vi "Facade.vi"(0 "Data In":T6, 2 "Display State In":T2, 3 "Container State":T5) -> (6 "Data Out":T6, 7 "Display State Out":T2, 8 "Action":T1)   [LabVIEW 2012, in "Hover Button.xctl"]
doc: "This facade vi is just a boolean button. The functionality associated with it allows the color properties of the button to change depending on whether the mouse is 'hovering' on the button."
uses:
  Hover Button.xctl
  Data.ctl
  <vilib>/_xctls/Container State.ctl
  State.ctl
  Button Colors.ctl
  Font Properties.ctl
  <vilib>/_xctls/Action.ctl
  Color Select.ctl
  <vilib>/_xctls/XControlSupport.lvlib
panel:
  in  "Boolean":bool
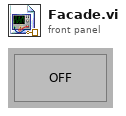
[diagram p1: front panel]
types:
  T1 = typedef "XControlSupport.lvlib/Action.ctl" = cluster{"Data Changed?":bool, "State Changed?":bool, "Action Name":string}
  T2 = typedef "Hover Button.xctl/State.ctl" = cluster{"On Text":string, "Off Text":string, "Current Color":T3, "Button Color":T3, "Hover Color":T3, "Show Boolean Text":bool, "Multiple Strings":bool, "Font":T4}
  T3 = typedef "Hover Button.xctl/Button Colors.ctl" = cluster{"On Color":u32, "Text Color":u32, "Off Color":u32}
  T4 = typedef "Hover Button.xctl/Font Properties.ctl" = cluster{"Font Name":string, "Size":u32, "Bold":bool, "Italic":bool, "Underline":bool, "Strikeout":bool, "Alignment":enum16{"Left", "Center", "Right"}}
  T5 = typedef "XControlSupport.lvlib/Container State.ctl" = cluster{"Indicator?":bool, "Run Mode?":bool, " Refnum":refnum<vi>}
  T6 = typedef "Hover Button.xctl/Data.ctl" = bool
  T7 = typedef "Hover Button.xctl/Color Select.ctl" = enum16{"Current Color", "Button Color", "Hover Color"}
  T8 = cluster{"Text Color":u32, "Background Color":u32}
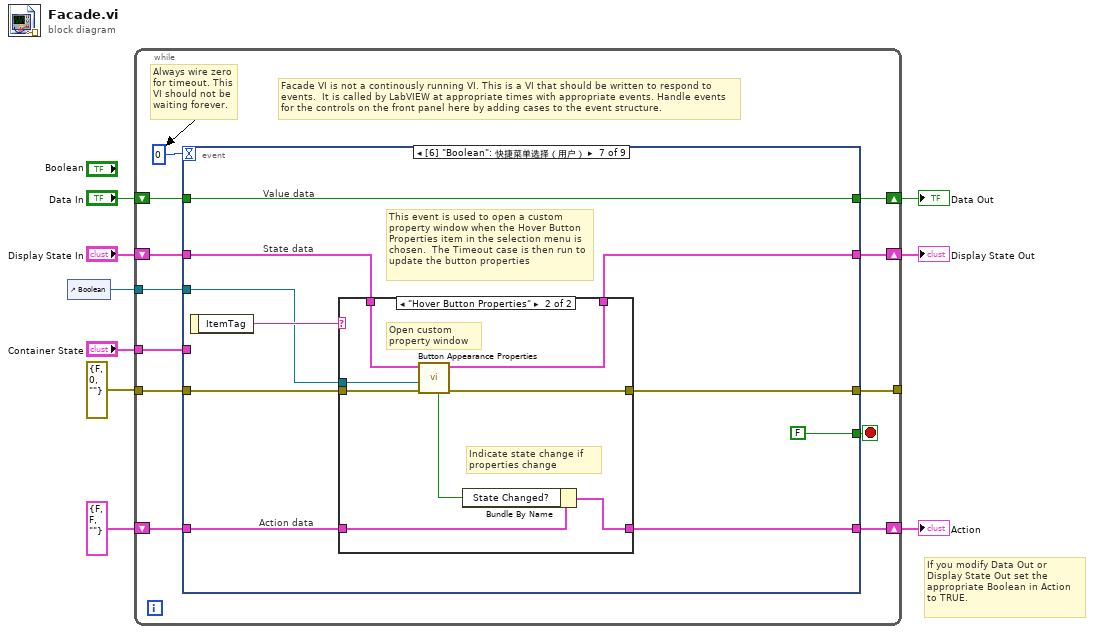
[diagram p0: block diagram]
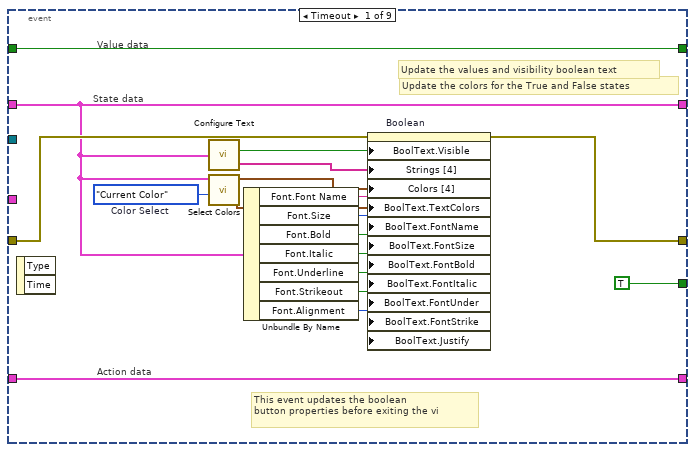
[diagram p2: hidden frame]
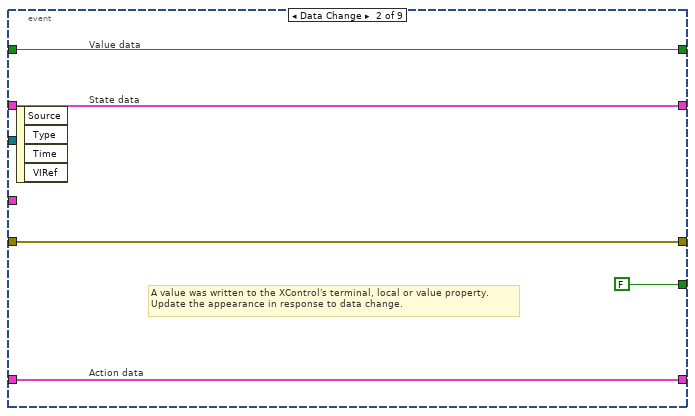
[diagram p3: hidden frame]
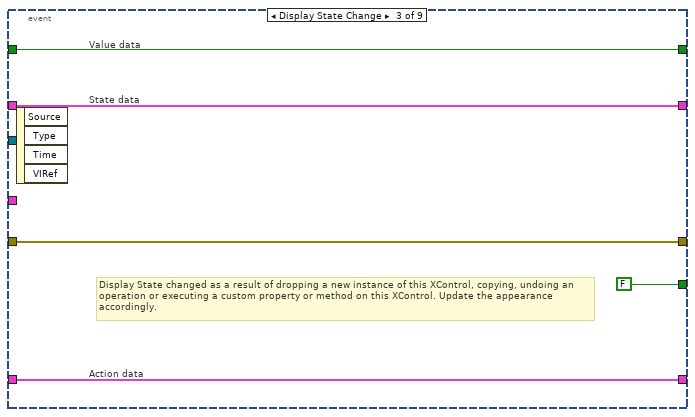
[diagram p4: hidden frame]
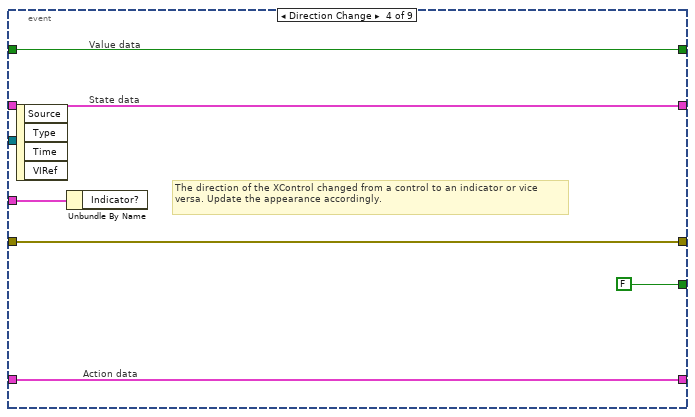
[diagram p5: hidden frame]
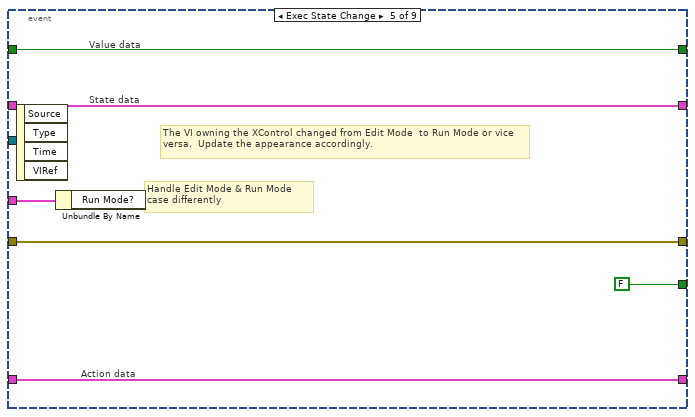
[diagram p6: hidden frame]
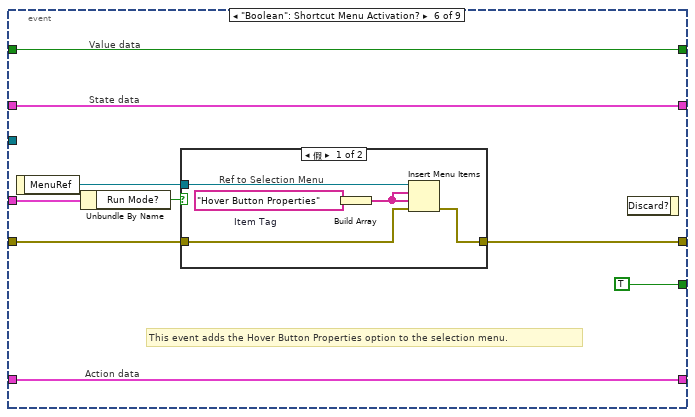
[diagram p7: hidden frame]
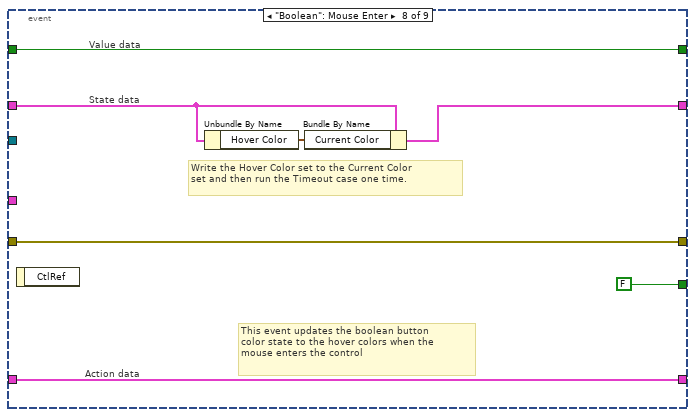
[diagram p10: hidden frame]
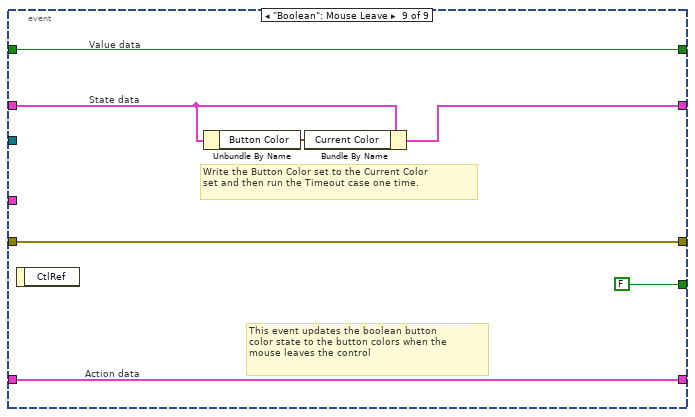
[diagram p11: hidden frame]
diagram:
  # "If you modify Data Out or\nDisplay State Out set the\nappropriate Boolean in Action\nto TRUE."
  n1 = control-ref of="Boolean"() -> (w1:refnum<vi>)
  n2 = while {
    shift-right: [w20] -> w6
    shift-left: "Display State In" -> [w21]
    tunnel: "Container State" -> [w17]
    shift-right: [w15] -> w9
    shift-left: "Data In" -> [w16]
    shift-right: [w13] -> w4
    shift-left: T1 {"Data Changed?"=FALSE, "State Changed?"=FALSE, "Action Name"=""} ("Action") -> [w14]
    tunnel: errorcluster {"status"=FALSE, "code"=0, "source"=""} ("Error In") -> [w12]
    tunnel: [w11] -> _
    tunnel: w1 -> [w10]
    stop <- w19 stop-if-true
    # "Facade VI is not a continously running VI. This is a VI that should be written to respond to events.  It is called by LabVIEW at appropriate times with appropriate events. Handle events for the controls on the front panel here by adding cases to the event structure."
    # "Always wire zero for timeout. This\nVI should not be waiting forever."
    n3 = event shown="[6] \"Boolean\": 快捷菜单选择（用户）" {
      selector: _ -> [_ _ _ _ _ _ _ _ _]
      dyn-events: _ -> [_ _ _ _ _ _ _ _ _]
      timeout: 0 -> [_ _ _ _ _ _ _ _ _]
      tunnel: w21 -> [w29 w44 w45 w54 w60 w67 w81 w101 w108]
      tunnel: [w29 w44 w45 w54 w60 w67 w80 w100 w107] -> w20
      tunnel: [TRUE FALSE FALSE FALSE FALSE TRUE FALSE FALSE FALSE] -> w19
      tunnel: w17 -> [_ _ _ w55 w61 w70 _ _ _]
      tunnel: w16 -> [w37 w43 w49 w53 w59 w66 w85 w104 w111]
      tunnel: [w37 w43 w49 w53 w59 w66 w85 w104 w111] -> w15
      tunnel: [w38 w42 w47 w52 w58 w65 w82 w103 w110] -> w13
      tunnel: w14 -> [w38 w42 w47 w52 w58 w65 w83 w103 w110]
      tunnel: w12 -> [w33 w40 w46 w50 w56 w63 w79 w98 w105]
      tunnel: [w30 w40 w46 w50 w56 w62 w78 w98 w105] -> w11
      tunnel: w10 -> [_ _ _ _ _ _ w77 _ _]
      event Timeout {
        w36 = Color_Select."Current Color"  # Color Select
        # "Action data"
        # "Value data"
        # "State data"
        # "Update the colors for the True and False states"
        # "Update the values and visibility boolean text"
        # "This event updates the boolean\nbutton properties before exiting the vi"
        n4 = event-data() -> ()  [unwired: 1 in, 2 out]
        n5 = call "Configure Text.vi"("Display State In"=w29) -> ("Show Boolean Text"=w35:bool, "Text Array"=w34:string[])
        n6 = call "Select Colors.vi"("Color Select"=w36, "State"=w29) -> ("Text Colors"=w31:T8, "Button Colors"=w32:cluster{"FG":u32, "BG":u32}[])  [unwired: 8 in]
        n7 = Unbundle By Name(w29) -> ("Font.Font Name"=w28:string, "Font.Size"=w27:u32, "Font.Bold"=w26:bool, "Font.Italic"=w25:bool, "Font.Underline"=w24:bool, "Font.Strikeout"=w23:bool, "Font.Alignment"=w22:enum16{"Left", "Center", "Right"})
        n8 = property on="Boolean" class="Bool (严格)"(error in=w33, "BoolText.Visible"=w35, "Strings [4]"=w34, "Colors [4]"=w32, "BoolText.TextColors"=w31, "BoolText.FontName"=w28, "BoolText.FontSize"=w27, "BoolText.FontBold"=w26, "BoolText.FontItalic"=w25, "BoolText.FontUnder"=w24, "BoolText.FontStrike"=w23, "BoolText.Justify"=w22) -> (error out=w30:errorcluster)  [unwired: 1 in, 1 out]
      }
      event Data Change {
        # "Action data"
        # "State data"
        # "Value data"
        # "A value was written to the XControl's terminal, local or value property.\nUpdate the appearance in response to data change."
        n9 = event-data() -> ()  [unwired: 1 in, 4 out]
      }
      event Display State Change {
        # "Action data"
        # "State data"
        # "Value data"
        # "Display State changed as a result of dropping a new instance of this XControl, copying, undoing an operation or executing a custom property or method on this XControl. Update the appearance accordingly."
        n10 = event-data() -> ()  [unwired: 1 in, 4 out]
      }
      event Direction Change {
        # "Action data"
        # "State data"
        # "Value data"
        # "The direction of the XControl changed from a control to an indicator or vice versa. Update the appearance accordingly."
        n11 = event-data() -> ()  [unwired: 1 in, 4 out]
        n12 = Unbundle By Name(w55) -> ()  [unwired: 1 out]
      }
      event Exec State Change {
        # "Action data"
        # "State data"
        # "Value data"
        # "The VI owning the XControl changed from Edit Mode  to Run Mode or vice versa.  Update the appearance accordingly."
        # "Handle Edit Mode & Run Mode\ncase differently"
        n13 = event-data() -> ()  [unwired: 1 in, 4 out]
        n14 = Unbundle By Name(w61) -> ()  [unwired: 1 out]
      }
      event "Boolean": Shortcut Menu Activation? {
        # "Action data"
        # "State data"
        # "Value data"
        # "This event adds the Hover Button Properties option to the selection menu."
        n15 = event-data() -> ("MenuRef"=w68:refnum<k9>)  [unwired: 1 in]
        n16 = Unbundle By Name(w70) -> ("Run Mode?"=w69:bool)
        n17 = case shown="假" w69 {
          tunnel: w68 -> [w73 _]
          tunnel: w63 -> [w72 w76]
          tunnel: [w71 w76] -> w62
          frame False {
            w74 = "Hover Button Properties"  # Item Tag
            # "Ref to Selection Menu"
            n18 = Build Array(w74) -> (w75:string[])
            n19 = Insert Menu Items(6:w72, 7:w75, 8:w75, 9:w73) -> (0:w71:errorcluster)  [unwired: 2 in, 2 out]
          }
          frame True {
            # "Do nothing"
          }
        }
        n20 = event-data() -> ()  [unwired: 2 in, 1 out]
      }
      event "Boolean": Shortcut Menu Selection (User) {
        # "Action data"
        # "State data"
        # "Value data"
        # "This event is used to open a custom property window when the Hover Button Properties item in the selection menu is chosen.  The Timeout case is then run to update the button properties"
        n21 = event-data() -> ("ItemTag"=w86:string)  [unwired: 1 in]
        n22 = case shown="\"Hover Button Properties\"" w86 {
          tunnel: w83 -> [w88 w97]
          tunnel: [w88 w96] -> w82
          tunnel: w81 -> [w89 w94]
          tunnel: [w89 w95] -> w80
          tunnel: w79 -> [w87 w92]
          tunnel: [w87 w91] -> w78
          tunnel: w77 -> [_ w90]
          frame Default {
            # "Do nothing"
          }
          frame "Hover Button Properties" {
            # "Indicate state change if properties change"
            # "Open custom\nproperty window"
            n23 = call "Button Appearance Properties.vi"("Error In"=w92, "Bool Refnum"=w90, "Display State In"=w94) -> ("Error Out"=w91:errorcluster, "Display State Out"=w95:T2, "Change"=w93:bool)  [unwired: 6 in]
            n24 = Bundle By Name(cluster=w97, "State Changed?"=w93) -> (w96:T1)
          }
        }
      }
      event "Boolean": Mouse Enter {
        # "Action data"
        # "State data"
        # "Value data"
        # "Write the Hover Color set to the Current Color\nset and then run the Timeout case one time."
        # "This event updates the boolean button\ncolor state to the hover colors when the\nmouse enters the control"
        n25 = event-data() -> ()  [unwired: 1 in, 1 out]
        n26 = Unbundle By Name(w101) -> ("Hover Color"=w102:T3)
        n27 = Bundle By Name(cluster=w101, "Current Color"=w102) -> (w100:T2)
      }
      event "Boolean": Mouse Leave {
        # "Action data"
        # "State data"
        # "Value data"
        # "This event updates the boolean button\ncolor state to the button colors when the\nmouse leaves the control"
        # "Write the Button Color set to the Current Color\nset and then run the Timeout case one time."
        n28 = event-data() -> ()  [unwired: 1 in, 1 out]
        n29 = Unbundle By Name(w108) -> ("Button Color"=w109:T3)
        n30 = Bundle By Name(cluster=w108, "Current Color"=w109) -> (w107:T2)
      }
    }
  }
  "Display State Out" <- w6
  "Data Out" <- w9
  "Action" <- w4
